vi "myFFT_abc2pseq.vi"(1 "C spec":cdb, 2 "B spec":cdb, 3 "A spec":cdb) -> (0 "p seq spec":cdb)   [LabVIEW 2024]
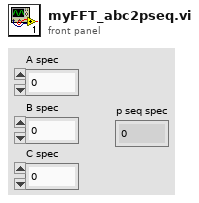
[diagram p1: front panel]
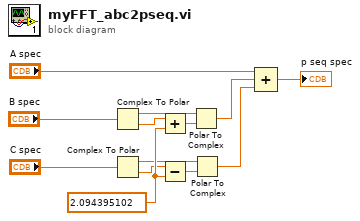
[diagram p0: block diagram]
diagram:
  w13 = 2.094395102
  n1 = Complex To Polar(r * e^(i*theta)="B spec") -> (r=w10:dbl, theta=w12:dbl)
  n2 = Complex To Polar(r * e^(i*theta)="C spec") -> (r=w8:dbl, theta=w11:dbl)
  n3 = Add(x=w12, y=w13) -> (x+y=w9:dbl)
  n4 = Subtract(x=w11, y=w13) -> (x-y=w7:dbl)
  n5 = Polar To Complex(1:w9, 2:w10) -> (0:w6:cdb)
  n6 = Polar To Complex(1:w7, 2:w8) -> (0:w5:cdb)
  n7 = Compound Arithmetic op=ADD("A spec", w6, w5) -> (→"p seq spec":cdb)
